vi "Open comm handler.vi"(8 "error in (no error)":errorcluster, 10 "timeout ms (1000)":i32=1000, 11 "WAMP Client in":refnum<class "WAMP Client.lvclass">) -> (0 "error out":errorcluster, 3 "WAMP Client out":refnum<class "WAMP Client.lvclass">)   [LabVIEW 2020, in "wamplv.lvlib" / "WAMP Client.lvclass"]
uses:
  WAMP Client.lvclass
  WAMP Client.lvclass/WAMP Client.ctl
  Private/Comm Handlers/ICommHandler/ICommHandler.lvclass
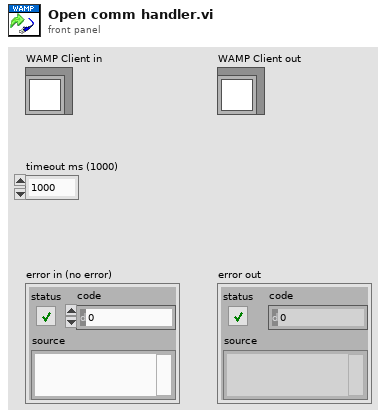
[diagram p1: front panel]
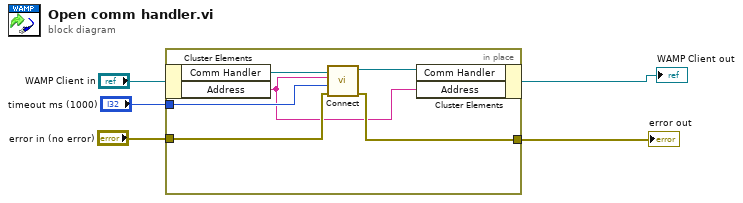
[diagram p0: block diagram]
diagram:
  n1 = in-place {
    in-place-border: "timeout ms (1000)" -> [w9]
    in-place-border: "error in (no error)" -> [w8]
    in-place-border: [w7] -> w1
    n2 = in-place-cluster #1("WAMP Client in") -> ("Comm Handler"=w11:refnum<class "ICommHandler.lvclass">, "Address"=w6:string)
    n3 = call-dynamic "Connect.vi"("error in"=w8, "timeout ms (1000)"=w9, "Address"=w6, "ICommHandler in"=w11) -> ("error out"=w7:errorcluster, "ICommHandler out"=w10:refnum<class "ICommHandler.lvclass">)  [unwired: 6 in]
    n4 = in-place-cluster #1("Comm Handler"=w10, "Address"=w6) -> (→"WAMP Client out":refnum<class "WAMP Client.lvclass">)
  }
  "error out" <- w1
